vi "CheckIfCurrentExceed.vi"(8 "error in (no error)":errorcluster, 9 "3P CurrentLimit":dbl caption="電流限制(A)", 10 "1P CurrentLimit":dbl caption="電流限制(A)", 11 "PW3390 in":refnum<class "PW3390.lvclass">) -> (0 "error out":errorcluster, 3 "PW3390 out":refnum<class "PW3390.lvclass">)   [LabVIEW 2024, in "PW3390 Actor.lvlib" / "PW3390.lvclass"]
uses:
  PW3390.lvclass
  C:/Program Files (x86)/National Instruments/LabVIEW 2024/vi.lib/ActorFramework/Actor/Actor.lvclass
  <vilib>/ActorFramework/Actor/Actor.lvclass/Actor.ctl
  PW3390.lvclass/PW3390.ctl
  MFActor/ActorMessage/MF Task Name.ctl
  <vilib>/ActorFramework/Actor/Actor.lvclass
  MFActor/ActorMessage/MFActorMsg.lvclass
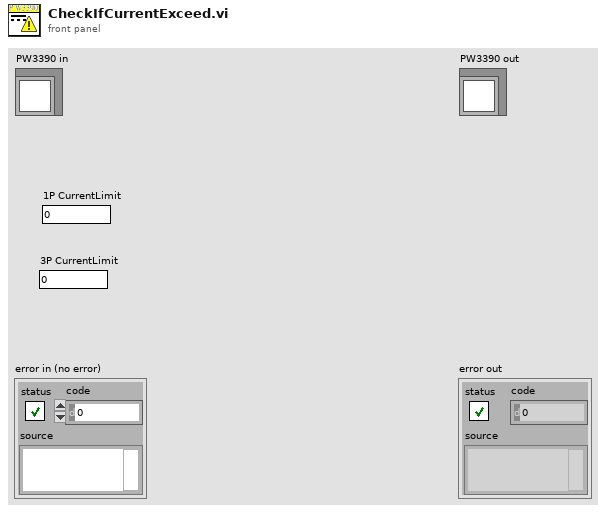
[diagram p1: front panel]
types:
  T1 = typedef "MF Task Name.ctl" = enum16{"DIChanged", "UpdateErrorCode", "SetTorque", "SetDriveTorque", "DataUpdated", "RunningTestProc", "StreamCtrl", "RunPID", "StopTest", "TCP Conn", "RefreshAutoUI", "ZeroAngle", "NestedActorLaunched", "NestedActorEnded", "ShowPsMsg"}
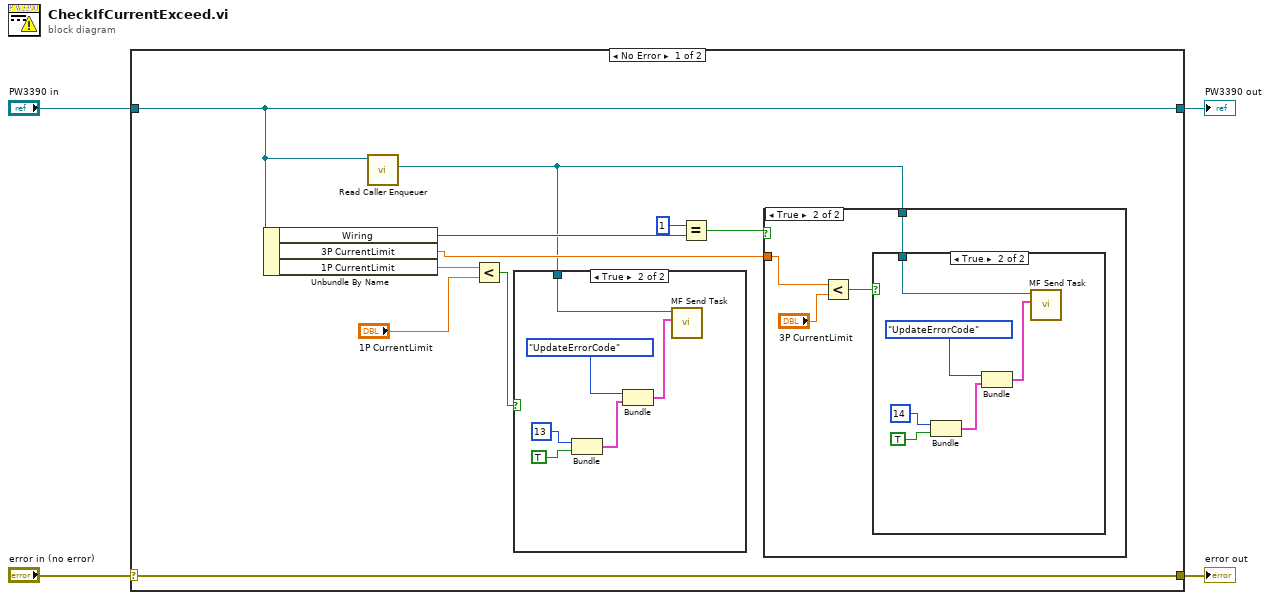
[diagram p0: block diagram]
diagram:
  n1 = case shown="No Error" "error in (no error)" {
    selector: "error in (no error)" -> [w14 w32]
    tunnel: [w14 w32] -> w3
    tunnel: [w7 w31] -> w1
    tunnel: "PW3390 in" -> [w7 w31]
    frame No Error {
      n2 = Unbundle By Name(w7) -> ("Wiring"=w12:u16, "3P CurrentLimit"=w8:dbl, "1P CurrentLimit"=w9:dbl)
      n3 = call <vilib>:"Read Caller Enqueuer.vi"("Actor"=w7) -> ("Caller Enqueuer"=w5:refnum<class "Message Enqueuer.lvclass">)  [unwired: 10 in]
      n4 = Less?(x=w9, y="1P CurrentLimit") -> (x < y?=w6:bool)
      n5 = case shown="True" w6 {
        tunnel: w5 -> [_ w20]
        frame False {
        }
        frame True {
          n6 = Bundle(13, TRUE) -> (w17:cluster{i32, bool})  [unwired: 1 in]
          n7 = Bundle("MF Msg Enum"=MF_Task_Name."UpdateErrorCode", w17) -> (w15:cluster{"MF Msg Enum":T1, cluster{i32, bool}})  [unwired: 1 in]
          n8 = call "MF Send Task.vi"("MsgType"=w15, "Message Enqueuer"=w20) -> ()  [unwired: 9 in, 1 out]
        }
      }
      n9 = Equal?(x=u16 1, y=w12) -> (x = y?=w10:bool)
      n10 = case shown="True" w10 {
        tunnel: w8 -> [_ w24]
        tunnel: w5 -> [_ w22]
        frame False {
        }
        frame True {
          n11 = Less?(x=w24, y="3P CurrentLimit") -> (x < y?=w21:bool)
          n12 = case shown="True" w21 {
            tunnel: w22 -> [_ w30]
            frame False {
            }
            frame True {
              n13 = Bundle(14, TRUE) -> (w27:cluster{i32, bool})  [unwired: 1 in]
              n14 = Bundle("MF Msg Enum"=MF_Task_Name."UpdateErrorCode", w27) -> (w25:cluster{"MF Msg Enum":T1, cluster{i32, bool}})  [unwired: 1 in]
              n15 = call "MF Send Task.vi"("MsgType"=w25, "Message Enqueuer"=w30) -> ()  [unwired: 9 in, 1 out]
            }
          }
        }
      }
    }
    frame Error {
    }
  }
  "error out" <- w3
  "PW3390 out" <- w1
